vi "报文编码.vi"(11 "data":T1 {"数组"."标识" items=["N"=1, "T"=2, "L"=3, "D"=4, "Z"=5, "M"=6, "hd"=7]; "数组"."污染物" items=["水温"=1, "浊度"=2, "DO"=3, "pH"=4, "ORP"=5, "比电导率"=6, "叶绿素a"=7, "氨氮"=8, "亚硝氮"=9, "硫化物"=10, "电压"=11, "温度"=12, "湿度"=13, "GPS经度"=14, "GPS纬度"=15, "BD经度"=16, "BD纬度"=17]; "数据类别" items=["水样数据"=0, "标样数据"=1, "零点核查数据"=2, "跨度核查数据"=3, "环境变量"=4, "水样数据补传"=16, "标样核查数据补传"=17, "零点核查数据补传"=18, "跨度核查数据补传"=19]}) -> (2 "数组":u8[](array[numeric]) format="%02xH", 3 "字符串":string)   [LabVIEW 2016, in "环境动力监测库.lvlib" / "NMEA.lvlib"]
uses:
  NMEA.lvlib
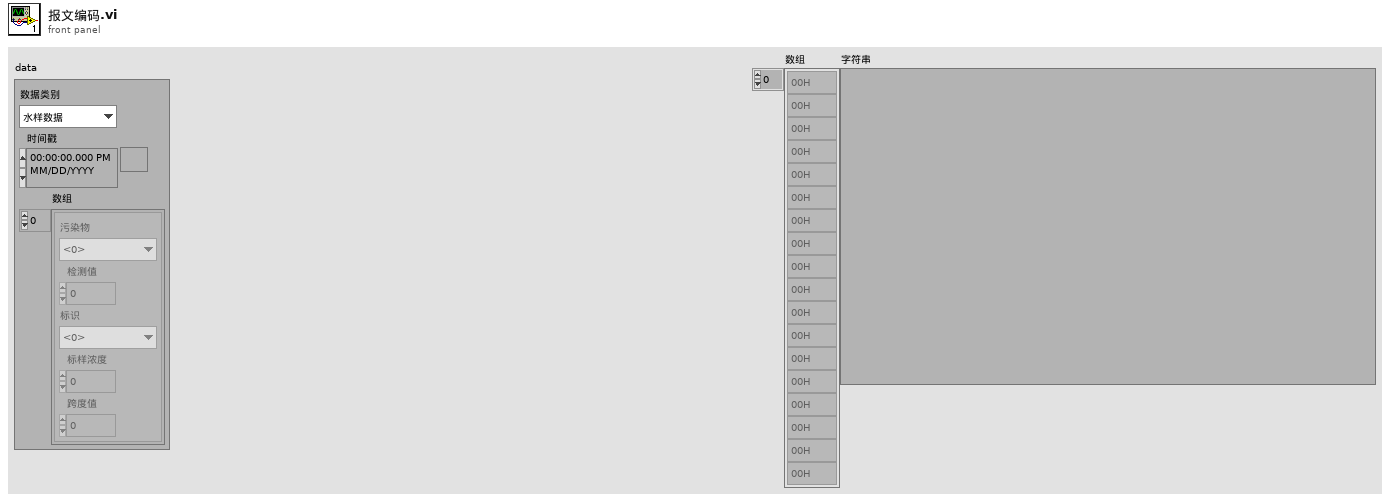
[diagram p1: front panel]
types:
  T1 = cluster{"数据类别":u16, "时间戳":timestamp, "数组":cluster{"污染物":u16, "检测值":dbl, "标识":u16, "标样浓度":dbl, "跨度值":dbl}[]}
  T2 = cluster{"污染物":u16, "检测值":dbl, "标识":u16, "标样浓度":dbl, "跨度值":dbl}[]
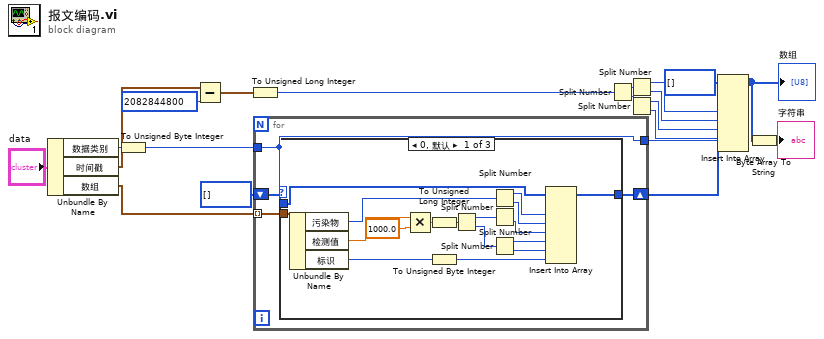
[diagram p0: block diagram]
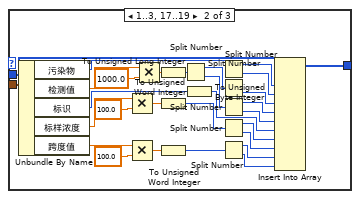
[diagram p2: hidden frame]
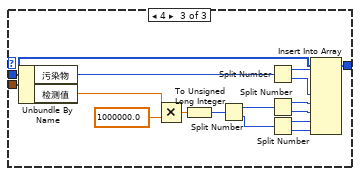
[diagram p3: hidden frame]
diagram:
  n1 = Unbundle By Name("data") -> ("数据类别"=w19:u16, "时间戳"=w17:timestamp, "数组"=w4:T2)
  n2 = To Unsigned Byte Integer(number=w19) -> (unsigned 8bit integer=w3:u8)
  n3 = Subtract(x=w17, y=2082844800) -> (x-y=w18:timestamp)
  n4 = To Unsigned Long Integer(number=w18) -> (unsigned 32bit integer=w14:u32)
  n5 = for {
    tunnel: w4 -> [w23] mode=indexing
    shift-right: [w21] -> w1
    shift-left: u8[] [] ("数组") -> [w22]
    tunnel: w3 -> [w24]
    tunnel: [w24] -> w2
    n6 = case shown="0, 默认" w24 {
      tunnel: w23 -> [w41 w70 w86]
      tunnel: w22 -> [w39 w68 w84]
      tunnel: [w26 w43 w77] -> w21
      frame 0, Default {
        n7 = Unbundle By Name(w41) -> ("污染物"=w40:u16, "检测值"=w36:dbl, "标识"=w28:u16)
        n8 = Multiply(x=w36, y=1000.0) -> (x*y=w37:dbl)
        n9 = To Unsigned Long Integer(number=w37) -> (unsigned 32bit integer=w34:u32)
        n10 = To Unsigned Byte Integer(number=w28) -> (unsigned 8bit integer=w27:u8)
        n11 = Split Number(x=w34) -> (hi(x)=w32:u16, lo(x)=w33:u16)
        n12 = Split Number(x=w40) -> (hi(x)=w25:u8, lo(x)=w38:u8)
        n13 = Split Number(x=w32) -> (lo(x)=w31:u8)  [unwired: 1 out]
        n14 = Split Number(x=w33) -> (hi(x)=w30:u8, lo(x)=w29:u8)
        n15 = Insert Into Array(array=w39, new element #1=w25, new element #2=w38, new element #3=w31, new element #4=w30, new element #5=w29, new element #6=w27) -> (w26:u8[])  [unwired: 1 in]
      }
      frame 1..3, 17..19 {
        n16 = Unbundle By Name(w70) -> ("污染物"=w69:u16, "检测值"=w65:dbl, "标识"=w57:u16, "标样浓度"=w53:dbl, "跨度值"=w49:dbl)
        n17 = Multiply(x=w53, y=100.0) -> (x*y=w55:dbl)
        n18 = Multiply(x=w49, y=100.0) -> (x*y=w51:dbl)
        n19 = Multiply(x=w65, y=1000.0) -> (x*y=w66:dbl)
        n20 = To Unsigned Long Integer(number=w66) -> (unsigned 32bit integer=w63:u32)
        n21 = To Unsigned Word Integer(number=w55) -> (unsigned 16bit integer=w50:u16)
        n22 = To Unsigned Word Integer(number=w51) -> (unsigned 16bit integer=w48:u16)
        n23 = Split Number(x=w63) -> (hi(x)=w61:u16, lo(x)=w62:u16)
        n24 = To Unsigned Byte Integer(number=w57) -> (unsigned 8bit integer=w56:u8)
        n25 = Split Number(x=w69) -> (hi(x)=w42:u8, lo(x)=w67:u8)
        n26 = Split Number(x=w61) -> (lo(x)=w60:u8)  [unwired: 1 out]
        n27 = Split Number(x=w62) -> (hi(x)=w59:u8, lo(x)=w58:u8)
        n28 = Split Number(x=w50) -> (hi(x)=w47:u8, lo(x)=w46:u8)
        n29 = Split Number(x=w48) -> (hi(x)=w45:u8, lo(x)=w44:u8)
        n30 = Insert Into Array(array=w68, new element #1=w42, new element #2=w67, new element #3=w60, new element #4=w59, new element #5=w58, new element #6=w56, new element #7=w47, new element #8=w46, new element #9=w45, new element #10=w44) -> (w43:u8[])  [unwired: 1 in]
      }
      frame 4 {
        n31 = Unbundle By Name(w86) -> ("污染物"=w85:u16, "检测值"=w82:dbl)
        n32 = Multiply(x=w82, y=1000000.0) -> (x*y=w83:dbl)
        n33 = To Unsigned Long Integer(number=w83) -> (unsigned 32bit integer=w80:u32)
        n34 = Split Number(x=w80) -> (hi(x)=w78:u16, lo(x)=w79:u16)
        n35 = Split Number(x=w85) -> (hi(x)=w71:u8, lo(x)=w72:u8)
        n36 = Split Number(x=w78) -> (hi(x)=w73:u8, lo(x)=w74:u8)
        n37 = Split Number(x=w79) -> (hi(x)=w75:u8, lo(x)=w76:u8)
        n38 = Insert Into Array(array=w84, new element #1=w71, new element #2=w72, new element #3=w73, new element #4=w74, new element #5=w75, new element #6=w76) -> (w77:u8[])  [unwired: 1 in]
      }
    }
  }
  n39 = Split Number(x=w14) -> (hi(x)=w13:u16, lo(x)=w12:u16)
  n40 = Split Number(x=w13) -> (hi(x)=w11:u8, lo(x)=w10:u8)
  n41 = Split Number(x=w12) -> (hi(x)=w9:u8, lo(x)=w8:u8)
  n42 = Insert Into Array(array=u8[] [] ("数组"), new element #1=w2, new element #2=w11, new element #3=w10, new element #4=w9, new element #5=w8, new element #6=w1) -> (w7:u8[])  [unwired: 1 in]
  "数组" <- w7
  n43 = Byte Array To String(unsigned byte array=w7) -> (string=→"字符串":string)
